vi "Create Default Hierarchy Table Rows.vi"(8 "Error in":errorcluster caption="Error in (no error)", 11 "Data":T1) -> (0 "Error out":errorcluster, 3 "OK":bool)   [LabVIEW 2018]
uses:
  TypeDef/Main - Handle Heirarchy Drag&Drop - Data.ctl
  Attach Param - Bool.vi
  <vilib>/httpClient/LabVIEWHTTPClient.lvlib
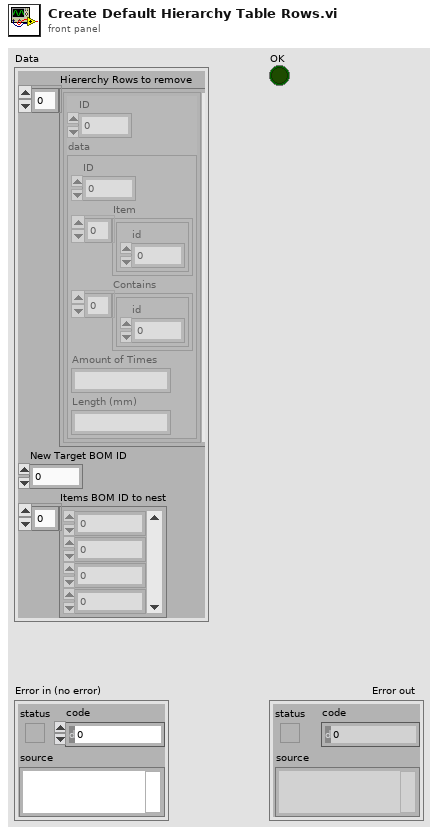
[diagram p1: front panel]
types:
  T1 = typedef "Main - Handle Heirarchy Drag&Drop - Data.ctl" = cluster{"Hiererchy Rows to remove":cluster{"ID":i32, "data":cluster{"ID":i32, "Item":cluster{"id":i32}[], "Contains":cluster{"id":i32}[], "Amount of Times":string, "Length (mm)":string}}[], "New Target BOM ID":i32, "Items BOM ID to nest":i32[]}
  T2 = typedef "LabVIEWHTTPClient.lvlib/ClientHandle.ctl" = refnum<k1>
  T3 = typedef "Param.ctl" = cluster{"Param":string, "Value":string}
  T4 = cluster{"Item":cluster{"id":i32}[], "Contains":cluster{"id":i32}[], "Amount of Times":string, "Length (mm)":string}
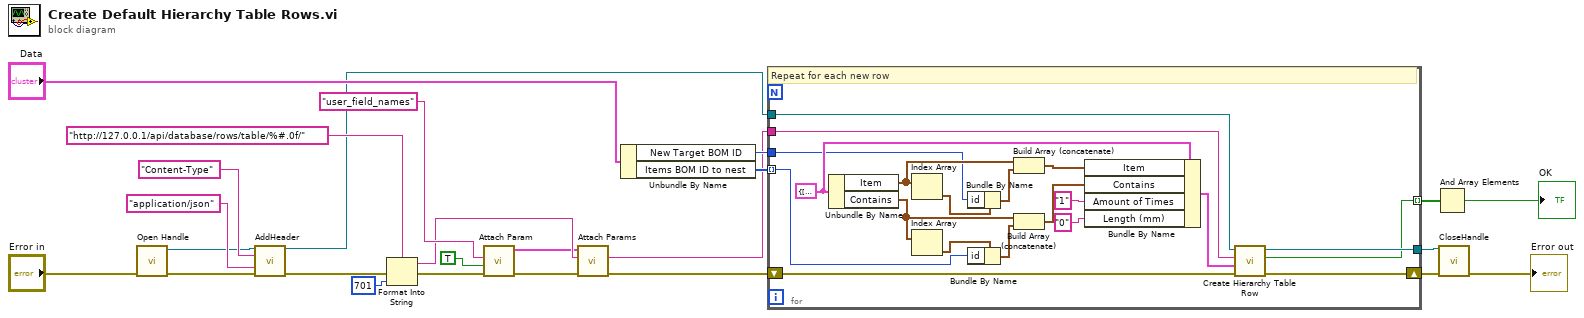
[diagram p0: block diagram]
diagram:
  n1 = call "Open Handle.vi"("error in (no error)"="Error in") -> ("error out"=w4:errorcluster, "Refnum out"=w6:T2)  [unwired: 9 in]
  n2 = call <vilib>:"AddHeader.vi"("client handle"=w6, "header"="Content-Type" ("value"), "value"="application/json", "error in (no error)"=w4) -> ("client handle out"=w5:T2, "error out"=w3:errorcluster)  [unwired: 10 in]
  n3 = Format Into String(format string="http://127.0.0.1/api/database/rows/table/%#.0f/" ("url"), error in=w3, u32 701 ("input 1")) -> (resulting string=w22:string, error out=w19:errorcluster)  [unwired: 1 in]
  n4 = call-poly "Attach Param.vi"("Error in"=w19, "Value"=TRUE, "Param Name"="user_field_names") -> ("Error out"=w20:errorcluster, "Params Array Out"=w21:T3[])  [unwired: 7 in]
  n5 = call "Attach Params.vi"("Error in"=w20, "URL"=w22, "Param array"=w21) -> ("Error out"=w13:errorcluster, "URL with params"=w12:string)  [unwired: 7 in]
  n6 = Unbundle By Name("Data") -> ("New Target BOM ID"=w15:i32, "Items BOM ID to nest"=w14:i32[])
  n7 = for {
    tunnel: w15 -> [w32]
    tunnel: w14 -> [w30] mode=indexing
    shift-right: [w40] -> w10
    shift-left: w13 -> [w45]
    tunnel: w5 -> [w44]
    tunnel: w12 -> [w43]
    tunnel: [w42] -> w11
    tunnel: [w41] -> w1 mode=indexing
    w37 = T4 {"Item"=[], "Contains"=[], "Amount of Times"="", "Length (mm)"=""} ("data")
    # "Repeat for each new row"
    n8 = Unbundle By Name(w37) -> ("Item"=w36:cluster{"id":i32}[], "Contains"=w28:cluster{"id":i32}[])
    n9 = Index Array(array=w36) -> (element=w35:cluster{"id":i32})  [unwired: 1 in]
    n10 = Index Array(array=w28) -> (element=w31:cluster{"id":i32})  [unwired: 1 in]
    n11 = Bundle By Name(cluster=w35, "id"=w32) -> (w34:cluster{"id":i32})
    n12 = Bundle By Name(cluster=w31, "id"=w30) -> (w26:cluster{"id":i32})
    n13 = Build Array (concatenate)(w36, w34) -> (w33:cluster{"id":i32}[])
    n14 = Build Array (concatenate)(w28, w26) -> (w27:cluster{"id":i32}[])
    n15 = Bundle By Name(cluster=w37, "Item"=w33, "Contains"=w27, "Amount of Times"="1", "Length (mm)"="0") -> (w39:T4)
    n16 = call "Create Hierarchy Table Row.vi"("error in (no error)"=w45, "data"=w39, "URL with params"=w43, "Refnum in"=w44) -> ("error out"=w40:errorcluster, "OK"=w41:bool, "Refnum out"=w42:T2)  [unwired: 5 in]
  }
  n17 = And Array Elements(Boolean array=w1) -> (logical AND=→"OK":bool)
  n18 = call <vilib>:"CloseHandle.vi"("client handle"=w11, "error in (no error)"=w10) -> ("error out"=→"Error out":errorcluster)  [unwired: 13 in]
